vi "Remove Broken Mappings.vi"(8 "error in":errorcluster, 11 "item ref in":T1 format="%.0x") -> (0 "error out":errorcluster, 3 "item ref out":T1 format="%.0x")   [LabVIEW 2027, in "Custom Device Serialization.lvlib"]
uses:
  Custom Device Serialization.lvlib
  <vilib>/NI VeriStand/Custom Device API/Custom Device Item Ref.ctl
  C:/NetCoreDLL/NationalInstruments.VeriStand.SystemStorage.dll
  NetCoreDLL/NationalInstruments.VeriStand.SystemStorage.dll
  C:/NetCoreDLL/NationalInstruments.VeriStand.SystemDefinitionAPI.dll
  NetCoreDLL/NationalInstruments.VeriStand.SystemDefinitionAPI.dll
  <vilib>/NI VeriStand/Custom Device API/Custom Device API.lvlib
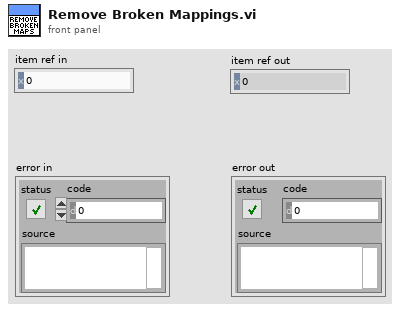
[diagram p1: front panel]
types:
  T1 = typedef "Custom Device API.lvlib/Custom Device Item Ref.ctl" = u64
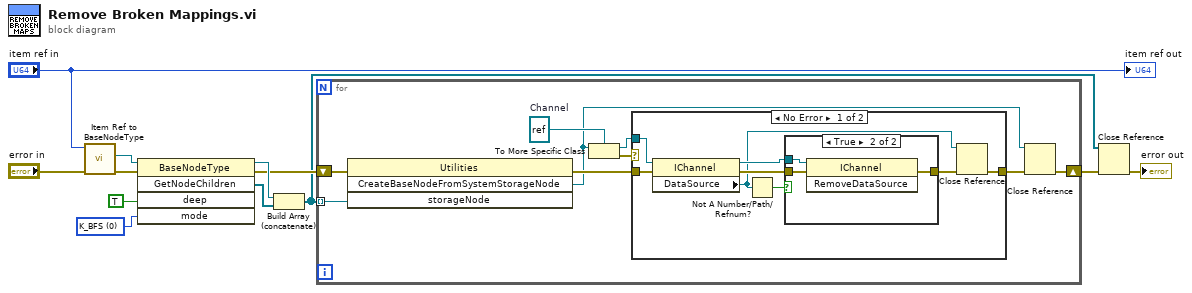
[diagram p0: block diagram]
diagram:
  w9 = 0 items=["K_BFS", "K_DFS", "K_CHILDONLY", "K_UP"] ("mode")
  n1 = call "Item Ref to BaseNodeType.vi"("error in (no error)"="error in", "item ref in"="item ref in") -> ("error out"=w5:errorcluster, "NationalInstruments.VeriStand.SystemStorage.BaseNodeType"=w8:refnum<k39>)  [unwired: 7 in, 1 out]
  n2 = invoke class="BaseNodeType" method="GetNodeChildren"(reference=w8, error in=w5, "deep"=TRUE, "mode"=w9) -> (reference out=w7:refnum<k39>, error out=w4:errorcluster, "GetNodeChildren"=w6:refnum<k39>[])  [unwired: 1 in, 2 out]
  n3 = Build Array (concatenate)(w7, w6) -> (w2:refnum<k39>[])
  n4 = for {
    tunnel: w2 -> [w21] mode=indexing
    shift-right: [w14] -> w3
    shift-left: w4 -> [w20]
    w18 = refnum<k39> refnum  # Channel
    n5 = invoke class="Utilities" method="CreateBaseNodeFromSystemStorageNode"(error in=w20, "storageNode"=w21) -> (error out=w16:errorcluster, "CreateBaseNodeFromSystemStorageNode"=w13:refnum<k39>)  [unwired: 2 in, 2 out]
    n6 = To More Specific Class(target class=w18, reference=w13) -> (specific class reference=w19:refnum<k39>, error out=w17:errorcluster)  [unwired: 1 in]
    n7 = case shown="No Error" w17 {
      tunnel: w19 -> [w26 _]
      tunnel: w16 -> [w29 w34]
      tunnel: [w23 w34] -> w15
      frame No Error {
        n8 = property class="IChannel"(reference=w26, error in=w29) -> (reference out=w25:refnum<k39>, error out=w27:errorcluster, "DataSource"=w22:refnum<k39>)
        n9 = Not A Number/Path/Refnum?(number/path/refnum=w22) -> (NaN/Path/Refnum?=w24:bool)
        n10 = case shown="True" w24 {
          tunnel: [w30 w33] -> w28
          tunnel: w27 -> [w30 w32]
          tunnel: w25 -> [_ w31]
          frame False {
          }
          frame True {
            n11 = invoke class="IChannel" method="RemoveDataSource"(reference=w31, error in=w32) -> (error out=w33:errorcluster)  [unwired: 1 in, 2 out]
          }
        }
        n12 = Close Reference(reference=w22, error in (no error)=w28) -> (error out=w23:errorcluster)
      }
      frame Error {
      }
    }
    n13 = Close Reference(reference=w13, error in (no error)=w15) -> (error out=w14:errorcluster)
  }
  n14 = Close Reference(reference=w2, error in (no error)=w3) -> (error out=→"error out":errorcluster)
  "item ref out" <- "item ref in"
